vi "Generate Gene.vi"(8 "error in":errorcluster, 11 "Character in":refnum<class "Character.lvclass">) -> (0 "error out":errorcluster, 3 "Character out":refnum<class "Character.lvclass">)   [LabVIEW 2016, in "Character.lvclass"]
uses:
  Character.lvclass
  Character.lvclass/Character.ctl
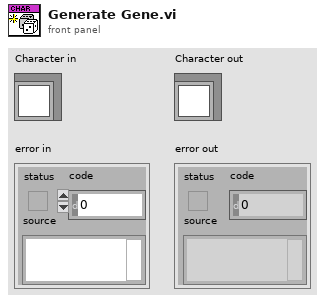
[diagram p1: front panel]
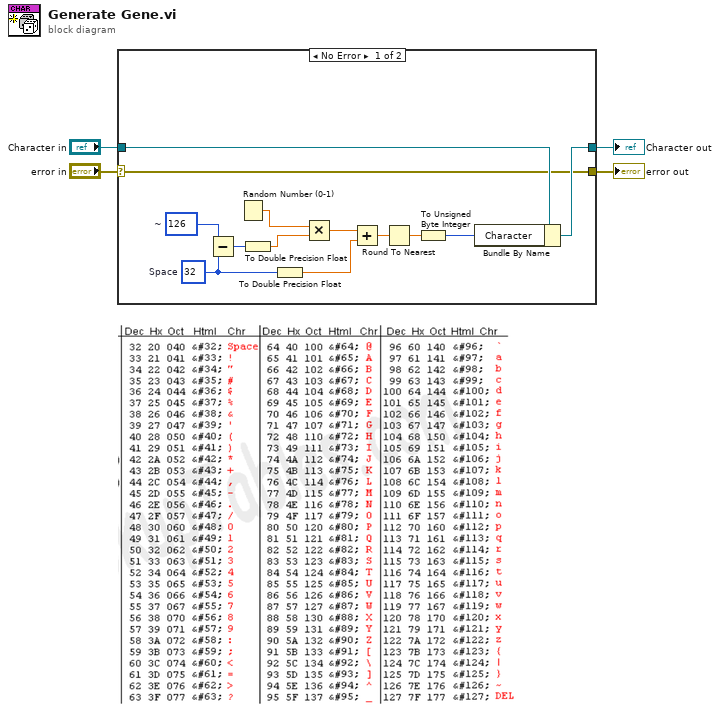
[diagram p0: block diagram]
diagram:
  n1 = case shown="No Error" "error in" {
    selector: "error in" -> [w5 w18]
    tunnel: "Character in" -> [w17 w19]
    tunnel: [w16 w19] -> w2
    tunnel: [w5 w18] -> w1
    frame No Error {
      w12 = u8 32  # Space
      w9 = u8 126  # ~
      n2 = Subtract(x=w9, y=w12) -> (x-y=w10:u8)
      n3 = Random Number (0-1)() -> (number: 0 to 1=w7:dbl)
      n4 = To Double Precision Float(number=w10) -> (double precision float=w8:dbl)
      n5 = To Double Precision Float(number=w12) -> (double precision float=w13:dbl)
      n6 = Multiply(x=w7, y=w8) -> (x*y=w11:dbl)
      n7 = Add(x=w11, y=w13) -> (x+y=w14:dbl)
      n8 = Round To Nearest(number=w14) -> (nearest integer value=w15:dbl)
      n9 = To Unsigned Byte Integer(number=w15) -> (unsigned 8bit integer=w6:u8)
      n10 = Bundle By Name(cluster=w17, "Character"=w6) -> (w16:refnum<class "Character.lvclass">)
    }
    frame Error {
    }
  }
  "error out" <- w1
  "Character out" <- w2
